vi "CalculatePhaseMagnitude.vi"(9 "phase reference channel":i32, 10 "previous phase":dbl[](array[numeric]), 11 "data":dbl[][](array[numeric])) -> (1 "last phase":dbl[](array[numeric]), 2 "Magnitude":dbl[][](array[numeric]), 3 "Phase":dbl[][](array[numeric]))   [LabVIEW 2013]
uses:
  <vilib>/Analysis/coordinate.llb/Angle Units.ctl
  <vilib>/Analysis/NI_AALPro.lvlib
  <vilib>/Analysis/NI_AAL_Angle.lvlib
panel:
  # "each row is I and then Q of one channel"
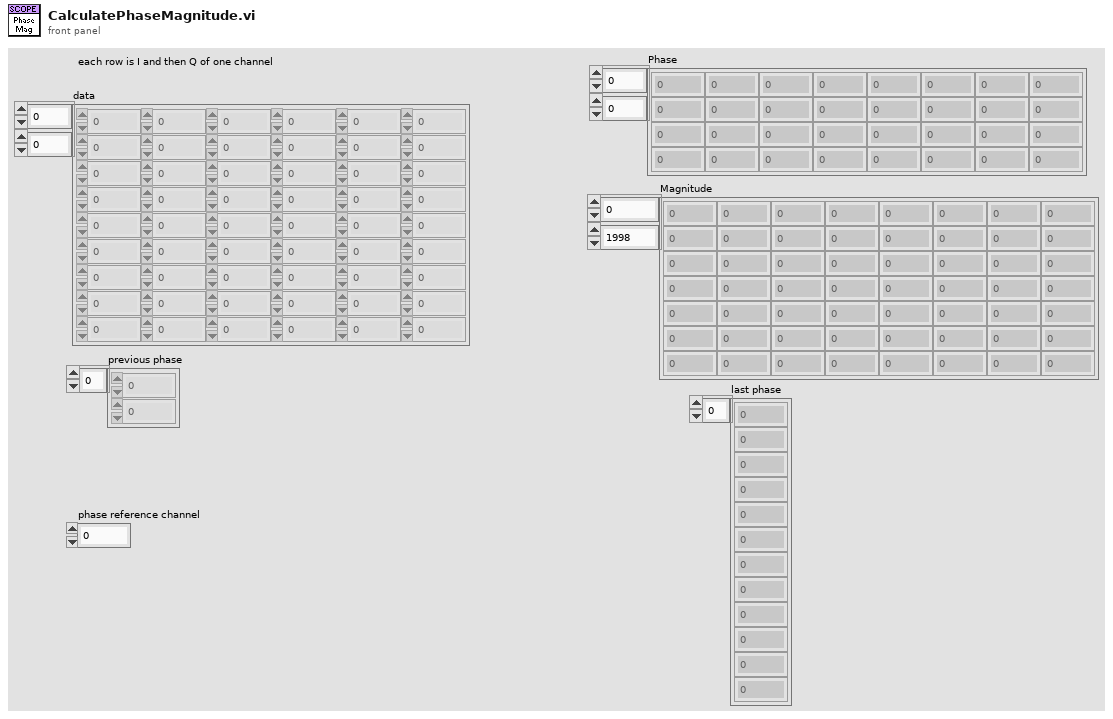
[diagram p1: front panel]
types:
  T1 = typedef "NI_AAL_Angle.lvlib/Angle Units.ctl" = i32
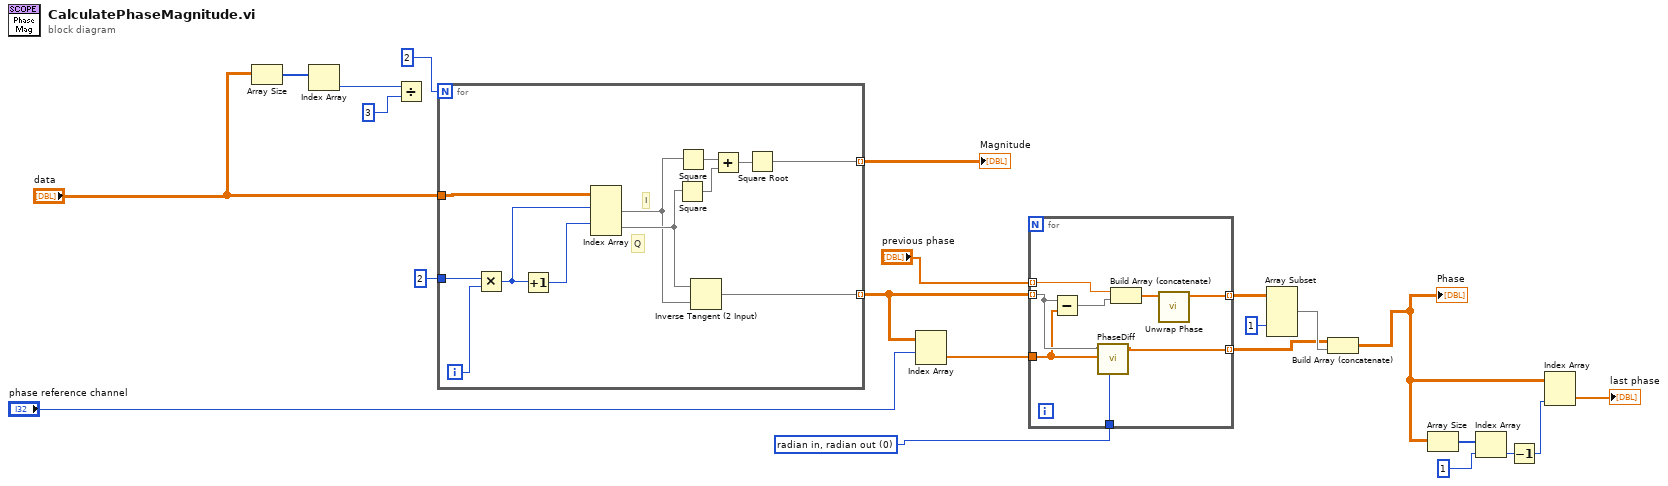
[diagram p0: block diagram]
diagram:
  w1 = T1 0 items=["radian in, radian out", "radian in, degree out", "degree in, degree out", "degree in, radian out"] ("angle units")
  n1 = Array Size(array="data") -> (size(s)=w10:i32[])
  n2 = Index Array(array=w10) -> (element=w9:i32)  [unwired: 1 in]
  n3 = Divide(x=w9, y=3) -> ()  [unwired: 1 out]
  n4 = for {
    N: 2 ("y") -> [_]
    tunnel: "data" -> [w34]
    tunnel: 2 ("y") -> [w33]
    tunnel: [w24] -> w21 mode=indexing
    tunnel: [w23] -> w12 mode=indexing
    i -> [w30]
    # "Q"
    # "I"
    n5 = Multiply(x=w33, y=w30) -> (x*y=w32:i32)
    n6 = Increment(x=w32) -> (x+1=w31:i32)
    n7 = Index Array(array=w34, index (row) #1=w32, index (row) #2=w31) -> (element #1=w25:dbl[], element #2=w26:dbl[])  [unwired: 2 in]
    n8 = Square(x=w26) -> (x^2=w28:dbl[])
    n9 = Square(x=w25) -> (x^2=w29:dbl[])
    n10 = Inverse Tangent (2 Input)(1:w25, 2:w26) -> (0:w23:dbl[])
    n11 = Add(x=w29, y=w28) -> (x+y=w27:dbl[])
    n12 = Square Root(x=w27) -> (sqrt(x)=w24:dbl[])
  }
  "Magnitude" <- w21
  n13 = Index Array(array=w12, index (row)="phase reference channel") -> (element=w11:dbl[])  [unwired: 1 in]
  n14 = for {
    tunnel: w12 -> [w38] mode=indexing
    tunnel: w11 -> [w37]
    tunnel: [w42] -> w4 mode=indexing
    tunnel: "previous phase" -> [w41] mode=indexing
    tunnel: [w36] -> w2 mode=indexing
    tunnel: w1 -> [w35]
    n15 = Subtract(x=w38, y=w37) -> (x-y=w39:dbl[])
    n16 = call "PhaseDiff.vi"("angle units"=w35, "Angle 2"=w37, "Angle 1"=w38) -> ("Absolute Angle Difference"=w36:dbl[])  [unwired: 5 in]
    n17 = Build Array (concatenate)(w41, w39) -> (w40:dbl[])
    n18 = call <vilib>:"Unwrap Phase.vi"("Phase"=w40) -> ("Unwrapped Phase"=w42:dbl[])  [unwired: 9 in, 1 out]
  }
  n19 = Array Subset(array=w4, index (col)=1 ("index")) -> (w3:dbl[][])  [unwired: 3 in]
  n20 = Build Array (concatenate)(w2, w3) -> (w13:dbl[][])
  "Phase" <- w13
  n21 = Array Size(array=w13) -> (size(s)=w18:i32[])
  n22 = Index Array(array=w18, index=1) -> (element=w17:i32)
  n23 = Decrement(x=w17) -> (x-1=w15:i32)
  n24 = Index Array(array=w13, index (col)=w15) -> (element=→"last phase":dbl[])  [unwired: 1 in]
